vi "Pressure Sensor-Remote.vi"() -> (1 "Scaled Value":u16 caption="Pressure")   [LabVIEW 2009]
uses:
  <vilib>/NXT/Block Support/NXT_InputPort.ctl
panel:
  in  "Input Port":T1 items=["Port 1", "Port 2", "Port 3", "Port 4"]
  # "mindsensors.com\nCopyright (c) 2009 by mindsensors.com\nEmail: info (<at>) mindsensors (<dot>) com\n\nThis program is free software. You can redistribute it and/or modify\nit under the terms of the GNU General Public License as published by\nthe Free Software Foundation; version 3 of the License.\nRead the license at: http://www.gnu.org/licenses/gpl.txt"
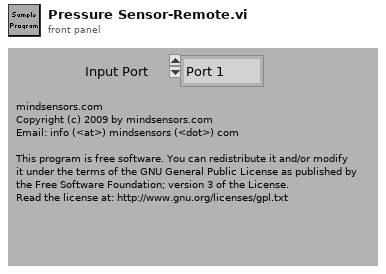
[diagram p1: front panel]
types:
  T1 = typedef "NXT_InputPort.ctl" = u8
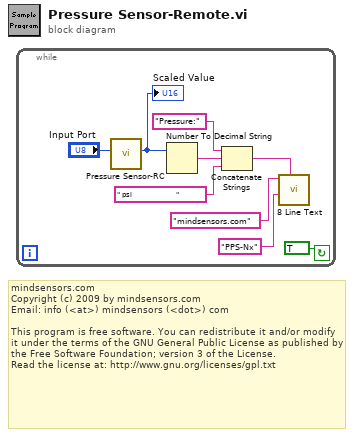
[diagram p0: block diagram]
diagram:
  # "mindsensors.com\nCopyright (c) 2009 by mindsensors.com\nEmail: info (<at>) mindsensors (<dot>) com\n\nThis program is free software. You can redistribute it and/or modify\nit under the terms of the GNU General Public License as published by\nthe Free Software Foundation; version 3 of the License.\nRead the license at: http://www.gnu.org/licenses/gpl.txt"
  n1 = while {
    stop <- TRUE continue-if-true
    n2 = call "Pressure Sensor-RC.vi"("Connection"="Input Port") -> ("Scaled Value"=w6:i16)  [unwired: 9 in, 1 out]
    "Scaled Value" <- w6
    n3 = Number To Decimal String(number=w6) -> (decimal integer string=w9:string)  [unwired: 1 in]
    n4 = Concatenate Strings("Pressure:" ("string"), w9, " psi                      " ("string")) -> (w2:string)
    n5 = call "8 Line Text.vi"("Line 5"=w2, "Line 3"="PPS-Nx", "Line 1"="mindsensors.com") -> ()  [unwired: 5 in]
  }
